vi "Automatic Teller Machine (ATM) SM based events.vi"() -> ()   [LabVIEW 2016]
doc: "This is the main VI of the ATM Machine simulation. This VI is developed using the design patterrn of Event based state machine."
uses:
  Controls/states.ctl
  Controls/Transaction Status.ctl
  Controls/UI Controls.ctl
  Controls/Module Data.ctl
  Controls/ATM Messages.ctl
  Controls/User Input Data.ctl
panel:
  in  "Module Data":T1={"UI Controls"={"ATM Messages"=refnum, "User Input"=refnum, "Right Buttons"=refnum, "Right Menu"=refnum, "Left Buttons"=refnum, "Left Menu"=refnum, "Card Simulator"=refnum, "Enter"=refnum}, "ATM Messages 2"={"Session terminate message"="Your session has been terminated\ndue to inactivity or menu selection.\nPlease take your card\n\nGoodbye!", "Welcome message"="Welcome to Acme bank.\nPlease insert your card\nand enter your account\nnumber in the User Input.\n\nPress Enter (E) when done.", "Deposit Message"="Please enter amount to deposit and press\nEnter (E) when done.", "Deposit Complete Message"="$ (Amount) Deposited", "Withdrawal Message"="Please enter amount to withdraw and press\nEnter (E) when done.", "Withdrawal Complete Message"="$ (Amount) Withdrawn", "Balance Inquiry Message"="Your Balance Is:\n$ (Balance amount from file)", "Account verification failed message"="Account information incorrect\nPlease Re-Enter Account Number.\nPress Enter (E) when done.", "Withdrawal failed message"="Insufficient funds in account\nplease check your balance\nand try again", "Card Inserted"="Card Inserted", "Main Menu message"="Welcome to Acme bank.\nFirst name, last Name (from file)\n\nplease select transaction\nby using the buttons."}, "User Input"="", "ATM Messages"="", "Acc. file path"=path "", "Accounts Data"=[], "User Input Data"={"Account No"="", "Amount"="", "Activity"=enum."Fast Cash $50"}, "Message"=""}
  in  "Enter":bool
  in  "User Input":string
  in  "Right Buttons":T6
  out "Right Menu":T7
  in  "Left Buttons":T6
  out "Left Menu":T7
  in  "Card Simulator":bool
  out "ATM Messages":string
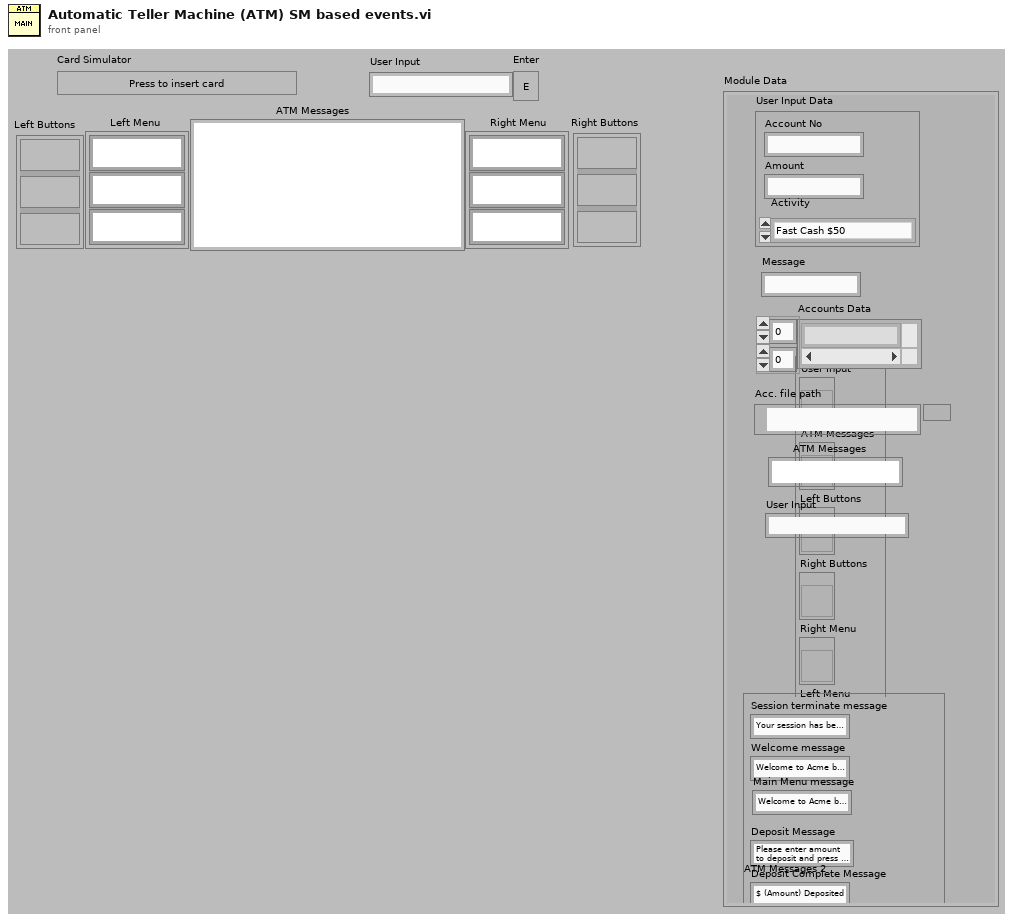
[diagram p1: front panel]
types:
  T1 = typedef "Module Data.ctl" = cluster{"UI Controls":T2, "ATM Messages 2":T3, "User Input":string, "ATM Messages":string, "Acc. file path":path, "Accounts Data":string[][], "User Input Data":T4, "Message":string}
  T2 = typedef "UI Controls.ctl" = cluster{"ATM Messages":refnum<vi>, "User Input":refnum<vi>, "Right Buttons":refnum<vi>, "Right Menu":refnum<vi>, "Left Buttons":refnum<vi>, "Left Menu":refnum<vi>, "Card Simulator":refnum<vi>, "Enter":refnum<vi>}
  T3 = typedef "ATM Messages.ctl" = cluster{"Session terminate message":string, "Welcome message":string, "Deposit Message":string, "Deposit Complete Message":string, "Withdrawal Message":string, "Withdrawal Complete Message":string, "Balance Inquiry Message":string, "Account verification failed message":string, "Withdrawal failed message":string, "Card Inserted":string, "Main Menu message":string}
  T4 = typedef "User Input Data.ctl" = cluster{"Account No":string, "Amount":string, "Activity":T5}
  T5 = typedef "Transaction Status.ctl" = enum16{"Fast Cash $50", "Withdrawal?", "Deposit?", "Account Number?"}
  T6 = cluster{"Func Button":bool, "Func Button 2":bool, "Func Button 3":bool}
  T7 = cluster{"RFS String":string, "RFS String 2":string, "RFS String 3":string}
  T8 = typedef "states.ctl" = enum16{"Deposit", "Enter Value", "Update Acc Number", "Make Correction in Acc No", "Wait for transaction", "Compare Account", "Read Accounts File", "Enter Account Number", "Wait for event", "Exit", "Initialize", "Insert ATM Card"}
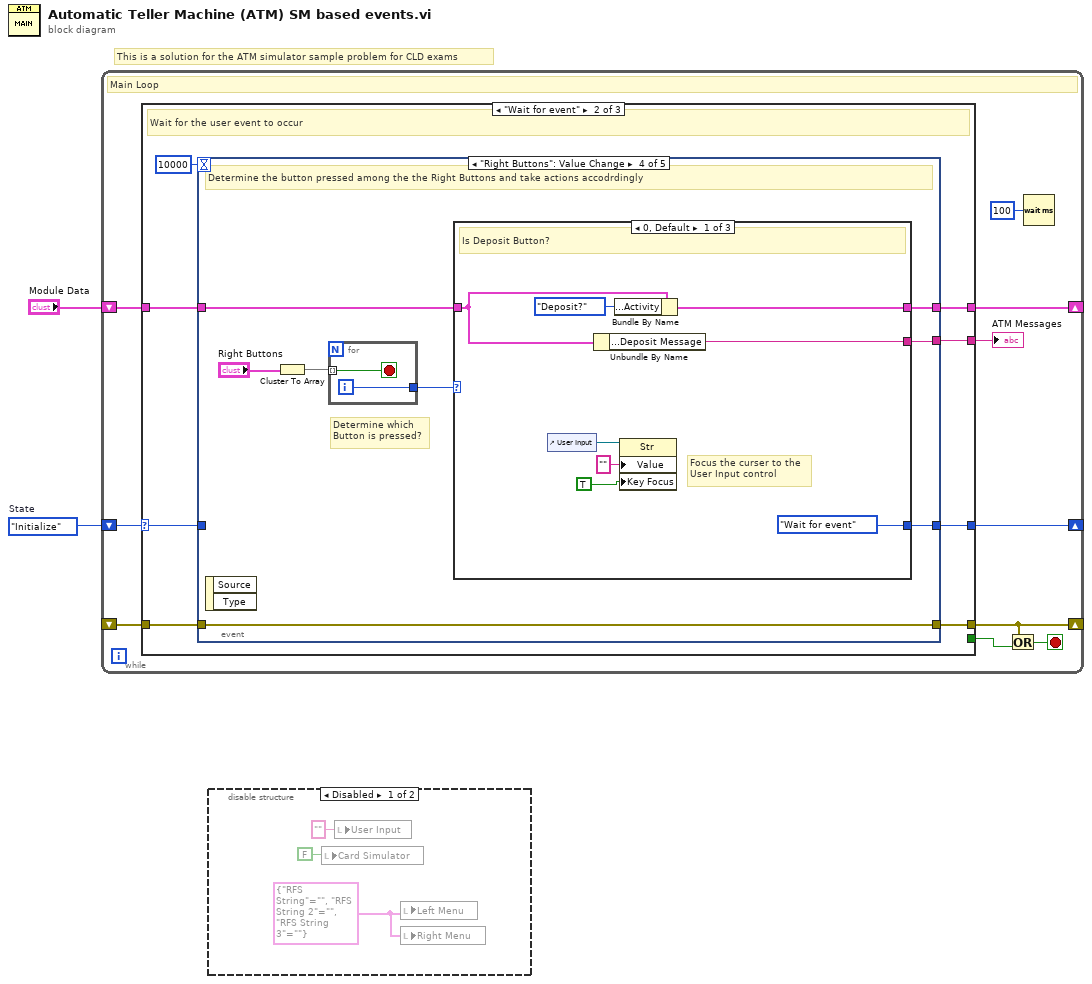
[diagram p0: block diagram]
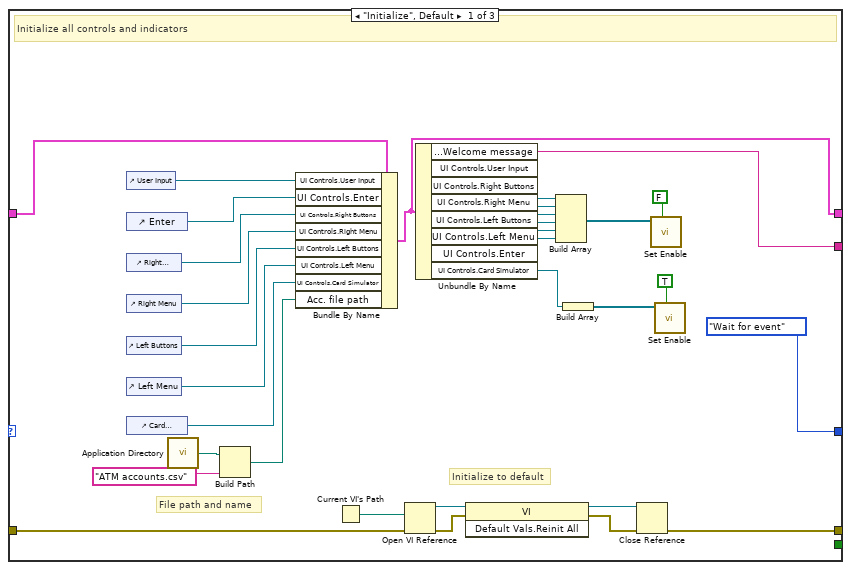
[diagram p3: hidden frame]
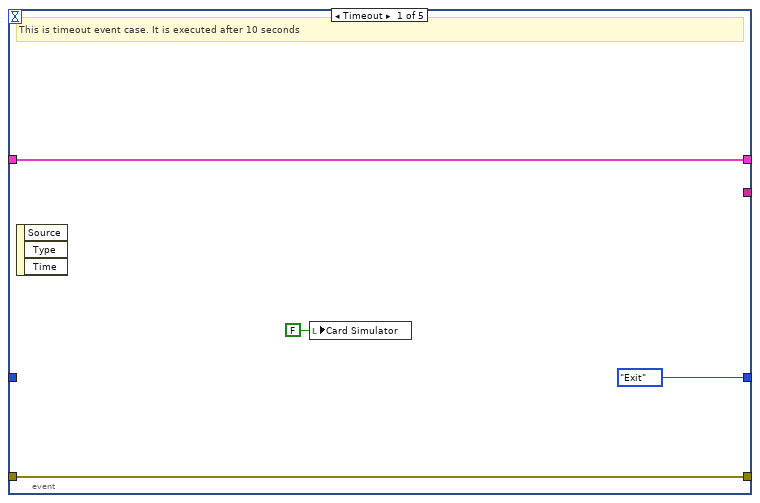
[diagram p4: hidden frame]
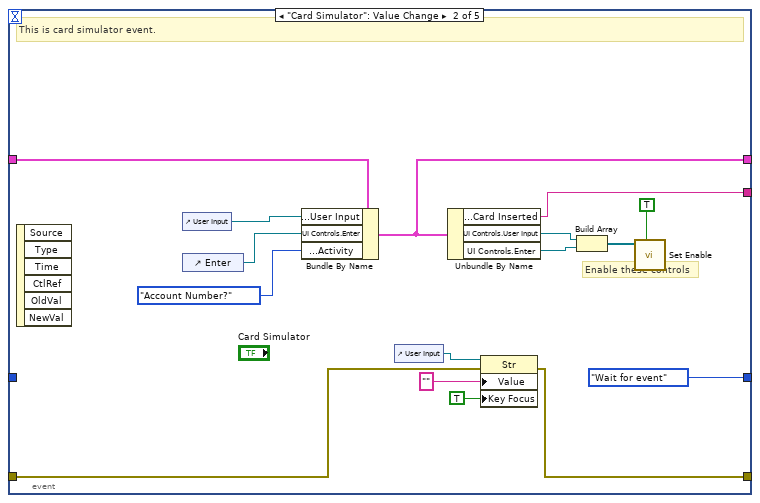
[diagram p5: hidden frame]
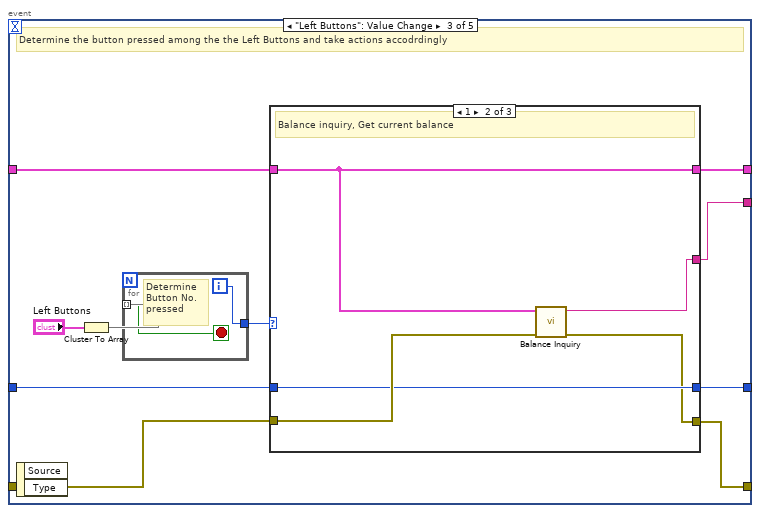
[diagram p6: hidden frame]
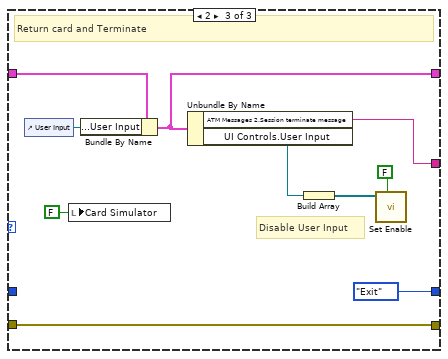
[diagram p8: hidden frame]
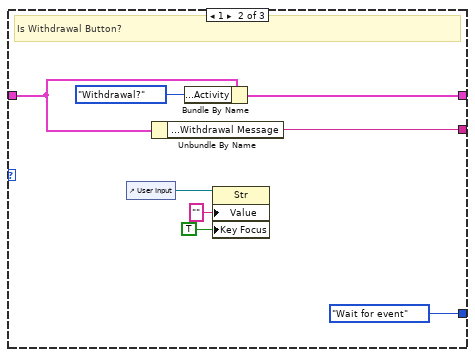
[diagram p9: hidden frame]
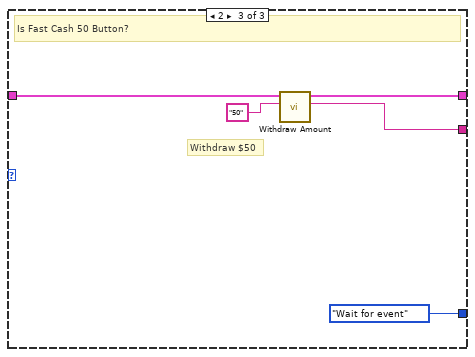
[diagram p10: hidden frame]
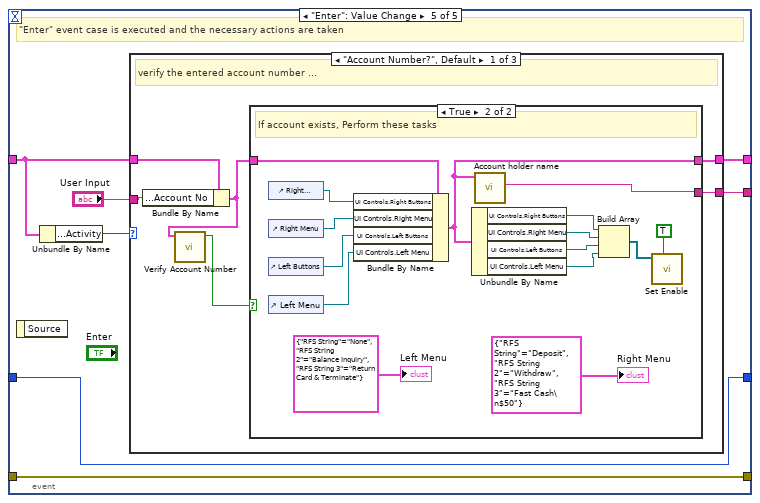
[diagram p11: hidden frame]
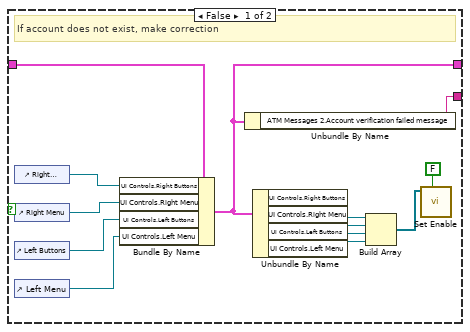
[diagram p12: hidden frame]
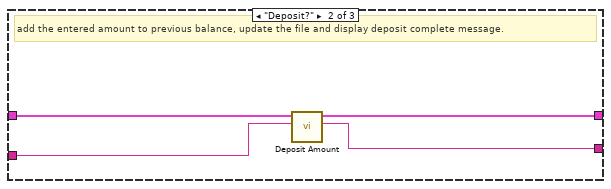
[diagram p13: hidden frame]
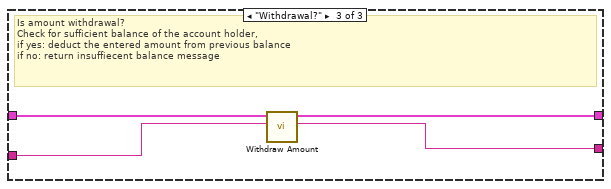
[diagram p14: hidden frame]
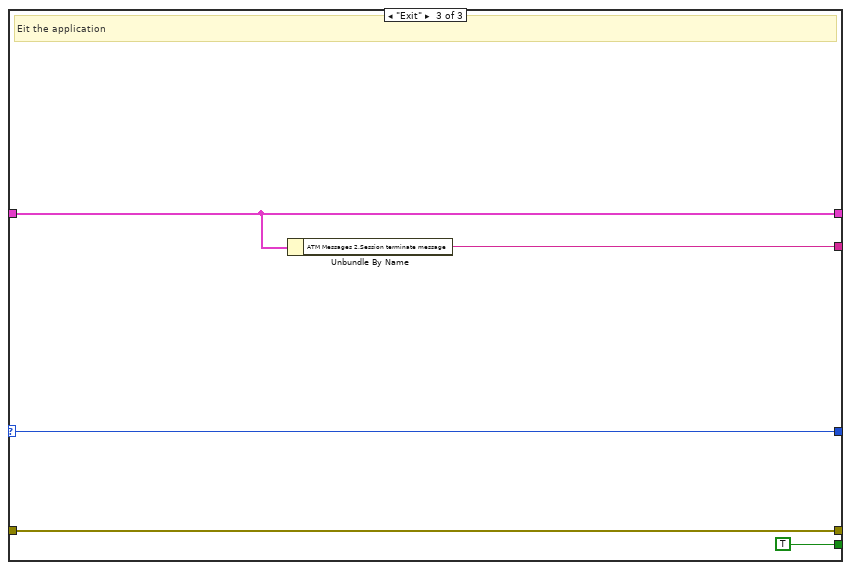
[diagram p15: hidden frame]
diagram:
  w1 = states."Initialize"  # State
  # "This is a solution for the ATM simulator sample problem for CLD exams"
  n1 = while {
    shift-right: [w12] -> _
    shift-left: "Module Data" -> [w11]
    shift-right: [w9] -> _
    shift-left: w1 -> [w10]
    shift-right: [w5] -> _
    shift-left: _ -> [w8]
    stop <- w3 stop-if-true
    # "Main Loop"
    n2 = case shown="\"Wait for event\"" w10 {
      selector: w10 -> [_ w49 w187]
      tunnel: [w28 w48 w183] -> w7
      tunnel: w11 -> [w33 w51 w184]
      tunnel: [w20 w45 w184] -> w12
      tunnel: [states."Wait for event" ("States") w50 w187] -> w9
      tunnel: [_ _ TRUE] -> w4
      tunnel: w8 -> [w17 w47 w185]
      tunnel: [w14 w46 w185] -> w5
      frame "Initialize", Default {
        # "Initialize to default"
        # "File path and name"
        # "Initialize all controls and indicators"
        n3 = control-ref of="User Input"() -> (w44:refnum<vi>)
        n4 = control-ref of="Enter"() -> (w43:refnum<vi>)
        n5 = control-ref of="Right Buttons"() -> (w42:refnum<vi>)
        n6 = control-ref of="Right Menu"() -> (w41:refnum<vi>)
        n7 = control-ref of="Left Buttons"() -> (w40:refnum<vi>)
        n8 = control-ref of="Left Menu"() -> (w39:refnum<vi>)
        n9 = control-ref of="Card Simulator"() -> (w25:refnum<vi>)
        n10 = call <vilib>:"Application Directory.vi"() -> ("Application Directory"=w23:path)
        n11 = Build Path(base path=w23, name or relative path="ATM accounts.csv") -> (appended path=w21:path)
        n12 = Bundle By Name(cluster=w33, "UI Controls.User Input"=w44, "UI Controls.Enter"=w43, "UI Controls.Right Buttons"=w42, "UI Controls.Right Menu"=w41, "UI Controls.Left Buttons"=w40, "UI Controls.Left Menu"=w39, "UI Controls.Card Simulator"=w25, "Acc. file path"=w21) -> (w20:T1)
        n13 = Current VI's Path() -> (path=w13:path)
        n14 = Open VI Reference(vi path=w13, error in (no error)=w17) -> (vi reference=w19:refnum<vi>, error out=w16:errorcluster)  [unwired: 4 in]
        n15 = Unbundle By Name(w20) -> ("ATM Messages 2.Welcome message"=w28:string, "UI Controls.User Input"=w38:refnum<vi>, "UI Controls.Right Buttons"=w37:refnum<vi>, "UI Controls.Right Menu"=w36:refnum<vi>, "UI Controls.Left Buttons"=w35:refnum<vi>, "UI Controls.Left Menu"=w34:refnum<vi>, "UI Controls.Enter"=w32:refnum<vi>, "UI Controls.Card Simulator"=w29:refnum<vi>)
        n16 = invoke class="VI" method="Default Vals.Reinit All"(reference=w19, error in=w16) -> (reference out=w18:refnum<vi>, error out=w15:errorcluster)  [unwired: 1 in, 1 out]
        n17 = Build Array(w38, w37, w36, w35, w34, w32) -> (w31:refnum<vi>[])
        n18 = Build Array(w29) -> (w30:refnum<vi>[])
        n19 = Close Reference(reference=w18, error in (no error)=w15) -> (error out=w14:errorcluster)
        n20 = call "Set Enable.vi"("Enable?"=FALSE, "UI Controls"=w31) -> ()  [unwired: 10 in]
        n21 = call "Set Enable.vi"("Enable?"=TRUE, "UI Controls"=w30) -> ()  [unwired: 10 in]
      }
      frame "Wait for event" {
        # "Wait for the user event to occur"
        n22 = event shown="[3] \"Right Buttons\": Value Change" {
          selector: _ -> [_ _ _ _ _]
          dyn-events: _ -> [_ _ _ _ _]
          timeout: 10000 -> [_ _ _ _ _]
          tunnel: w51 -> [w55 w69 w79 w106 w136]
          tunnel: [states."Exit" ("States") states."Wait for event" ("States") w75 w103 w135] -> w50
          tunnel: w49 -> [_ _ w74 _ w135]
          tunnel: [_ w64 w77 w105 w134] -> w48
          tunnel: w47 -> [w54 w57 w78 w110 w137]
          tunnel: [w54 w58 w73 w110 w137] -> w46
          tunnel: [w55 w62 w76 w104 w139] -> w45
          event Timeout {
            # "This is timeout event case. It is executed after 10 seconds"
            n23 = event-data() -> ()  [unwired: 1 in, 3 out]
            n24 = local write "Card Simulator"(FALSE ("Card Simulator")) -> ()
          }
          event "Card Simulator": Value Change {
            # "Enable these controls"
            # "This is card simulator event."
            n25 = event-data() -> ()  [unwired: 1 in, 6 out]
            n26 = control-ref of="User Input"() -> (w72:refnum<vi>)
            n27 = control-ref of="Enter"() -> (w71:refnum<vi>)
            n28 = Bundle By Name(cluster=w69, "UI Controls.User Input"=w72, "UI Controls.Enter"=w71, "User Input Data.Activity"=Transaction_Status."Account Number?" ("User Input Data.Transactions")) -> (w62:T1)
            n29 = control-ref of="User Input"() -> (w61:refnum<vi>)
            n30 = Unbundle By Name(w62) -> ("ATM Messages 2.Card Inserted"=w64:string, "UI Controls.User Input"=w68:refnum<vi>, "UI Controls.Enter"=w67:refnum<vi>)
            n31 = property class="Str"(reference=w61, error in=w57, "Value"="", "Key Focus"=TRUE) -> (error out=w58:errorcluster)  [unwired: 1 out]
            n32 = Build Array(w68, w67) -> (w66:refnum<vi>[])
            n33 = call "Set Enable.vi"("Enable?"=TRUE, "UI Controls"=w66) -> ()  [unwired: 10 in]
          }
          event "Left Buttons": Value Change {
            # "Determine the button pressed among the the Left Buttons and take actions accodrdingly"
            n34 = event-data() -> ()  [unwired: 1 in, 2 out]
            n35 = Cluster To Array(cluster="Left Buttons") -> (array=w81:bool[])
            n36 = for {
              tunnel: w81 -> [w84] mode=indexing
              tunnel: [w83] -> w80
              i -> [w83]
              stop <- w84 stop-if-true
              # "Determine\nButton No. \npressed"
            }
            n37 = case shown="1" w80 {
              tunnel: w79 -> [w87 w90 w101]
              tunnel: w78 -> [w85 w92 w98]
              tunnel: [_ w91 w93] -> w77
              tunnel: [w87 w90 w97] -> w76
              tunnel: [w86 w89 states."Exit" ("States")] -> w75
              tunnel: w74 -> [w86 w89 _]
              tunnel: [w85 w88 w98] -> w73
              frame 0, Default {
                # "Do nothing, this button is for\nfuture use."
              }
              frame 1 {
                # "Balance inquiry, Get current balance"
                n38 = call "Balance Inquiry.vi"("error in (no error)"=w92, "Module Data"=w90) -> ("error out"=w88:errorcluster, "Balance"=w91:string)  [unwired: 8 in]
              }
              frame 2 {
                # "Disable User Input"
                # "Return card and Terminate"
                n39 = control-ref of="User Input"() -> (w100:refnum<vi>)
                n40 = local write "Card Simulator"(FALSE ("Card Simulator")) -> ()
                n41 = Bundle By Name(cluster=w101, "UI Controls.User Input"=w100) -> (w97:T1)
                n42 = Unbundle By Name(w97) -> ("ATM Messages 2.Session terminate message"=w93:string, "UI Controls.User Input"=w96:refnum<vi>)
                n43 = Build Array(w96) -> (w95:refnum<vi>[])
                n44 = call "Set Enable.vi"("Enable?"=FALSE, "UI Controls"=w95) -> ()  [unwired: 10 in]
              }
            }
          }
          event "Right Buttons": Value Change {
            # "Determine which\nButton is pressed?"
            # "Determine the button pressed among the the Right Buttons and take actions accodrdingly"
            n45 = event-data() -> ()  [unwired: 1 in, 2 out]
            n46 = Cluster To Array(cluster="Right Buttons") -> (array=w108:bool[])
            n47 = for {
              tunnel: w108 -> [w132] mode=indexing
              tunnel: [w133] -> w107
              i -> [w133]
              stop <- w132 stop-if-true
            }
            n48 = case shown="0, Default" w107 {
              tunnel: w106 -> [w116 w124 w130]
              tunnel: [w117 w125 w127] -> w105
              tunnel: [w115 w123 w128] -> w104
              tunnel: [states."Wait for event" ("States") states."Wait for event" ("States") states."Wait for event" ("States")] -> w103
              frame 0, Default {
                # "Focus the curser to the\nUser Input control"
                # "Is Deposit Button?"
                n49 = control-ref of="User Input"() -> (w114:refnum<vi>)
                n50 = Unbundle By Name(w116) -> ("ATM Messages 2.Deposit Message"=w117:string)
                n51 = Bundle By Name(cluster=w116, "User Input Data.Activity"=Transaction_Status."Deposit?") -> (w115:T1)
                n52 = property class="Str"(reference=w114, "Value"="", "Key Focus"=TRUE) -> ()  [unwired: 1 in, 2 out]
              }
              frame 1 {
                # "Is Withdrawal Button?"
                n53 = control-ref of="User Input"() -> (w121:refnum<vi>)
                n54 = Unbundle By Name(w124) -> ("ATM Messages 2.Withdrawal Message"=w125:string)
                n55 = Bundle By Name(cluster=w124, "User Input Data.Activity"=Transaction_Status."Withdrawal?" ("Transactions")) -> (w123:T1)
                n56 = property class="Str"(reference=w121, "Value"="", "Key Focus"=TRUE) -> ()  [unwired: 1 in, 2 out]
              }
              frame 2 {
                # "Withdraw $50"
                # "Is Fast Cash 50 Button?"
                n57 = call "Withdraw Amount.vi"("User Input"="50", "Module Data in"=w130) -> ("Withdrawal Complete Message"=w127:string, "Module Data out"=w128:T1)  [unwired: 8 in]
              }
            }
          }
          event "Enter": Value Change {
            # "\"Enter\" event case is executed and the necessary actions are taken"
            n58 = event-data() -> ()  [unwired: 1 in, 1 out]
            n59 = Unbundle By Name(w136) -> ("User Input Data.Activity"=w140:T5)
            n60 = case shown="\"Account Number?\", Default" w140 {
              tunnel: w136 -> [w144 w176 w180]
              tunnel: [w143 w175 w182] -> w139
              tunnel: "User Input" -> [w146 w177 w179]
              tunnel: [w142 w178 w181] -> w134
              frame "Account Number?", Default {
                # "verify the entered account number ..."
                n61 = Bundle By Name(cluster=w144, "User Input Data.Account No"=w146) -> (w141:T1)
                n62 = call "Verify Account Number.vi"("Module Data"=w141) -> ("Is account?"=w145:bool)  [unwired: 6 in, 4 out]
                n63 = case shown="True" w145 {
                  tunnel: [w148 w161] -> w143
                  tunnel: w141 -> [w149 w174]
                  tunnel: [w159 w160] -> w142
                  frame False {
                    # "If account does not exist, make correction"
                    n64 = control-ref of="Right Buttons"() -> (w152:refnum<vi>)
                    n65 = control-ref of="Right Menu"() -> (w151:refnum<vi>)
                    n66 = control-ref of="Left Buttons"() -> (w150:refnum<vi>)
                    n67 = control-ref of="Left Menu"() -> (w147:refnum<vi>)
                    n68 = Bundle By Name(cluster=w149, "UI Controls.Right Buttons"=w152, "UI Controls.Right Menu"=w151, "UI Controls.Left Buttons"=w150, "UI Controls.Left Menu"=w147) -> (w148:T1)
                    n69 = Unbundle By Name(w148) -> ("ATM Messages 2.Account verification failed message"=w159:string)
                    n70 = Unbundle By Name(w148) -> ("UI Controls.Right Buttons"=w158:refnum<vi>, "UI Controls.Right Menu"=w157:refnum<vi>, "UI Controls.Left Buttons"=w156:refnum<vi>, "UI Controls.Left Menu"=w155:refnum<vi>)
                    n71 = Build Array(w158, w157, w156, w155) -> (w154:refnum<vi>[])
                    n72 = call "Set Enable.vi"("Enable?"=FALSE, "UI Controls"=w154) -> ()  [unwired: 10 in]
                  }
                  frame True {
                    # "If account exists, Perform these tasks"
                    n73 = control-ref of="Right Buttons"() -> (w173:refnum<vi>)
                    n74 = control-ref of="Right Menu"() -> (w172:refnum<vi>)
                    n75 = control-ref of="Left Buttons"() -> (w171:refnum<vi>)
                    n76 = control-ref of="Left Menu"() -> (w170:refnum<vi>)
                    n77 = Bundle By Name(cluster=w174, "UI Controls.Right Buttons"=w173, "UI Controls.Right Menu"=w172, "UI Controls.Left Buttons"=w171, "UI Controls.Left Menu"=w170) -> (w161:T1)
                    n78 = Unbundle By Name(w161) -> ("UI Controls.Right Buttons"=w167:refnum<vi>, "UI Controls.Right Menu"=w166:refnum<vi>, "UI Controls.Left Buttons"=w165:refnum<vi>, "UI Controls.Left Menu"=w164:refnum<vi>)
                    n79 = call "Account holder name.vi"("Module Data in"=w161) -> ("Withdrawal Complete Message"=w160:string)  [unwired: 10 in]
                    n80 = Build Array(w167, w166, w165, w164) -> (w163:refnum<vi>[])
                    n81 = call "Set Enable.vi"("Enable?"=TRUE, "UI Controls"=w163) -> ()  [unwired: 10 in]
                    "Left Menu" <- T7 {"RFS String"="None", "RFS String 2"="Balance Inquiry", "RFS String 3"="Return Card & Terminate"} ("Left Menu")
                    "Right Menu" <- T7 {"RFS String"="Deposit", "RFS String 2"="Withdraw", "RFS String 3"="Fast Cash\n$50"} ("Right Menu")
                  }
                }
              }
              frame "Deposit?" {
                # "add the entered amount to previous balance, update the file and display deposit complete message."
                n82 = call "Deposit Amount.vi"("User Input"=w177, "Module Data in"=w176) -> ("Deposit Complete Message"=w178:string, "Module Data out"=w175:T1)  [unwired: 8 in]
              }
              frame "Withdrawal?" {
                # "Is amount withdrawal?\nCheck for sufficient balance of the account holder, \nif yes: deduct the entered amount from previous balance\nif no: return insuffiecent balance message"
                n83 = call "Withdraw Amount.vi"("User Input"=w179, "Module Data in"=w180) -> ("Withdrawal Complete Message"=w181:string, "Module Data out"=w182:T1)  [unwired: 8 in]
              }
            }
          }
        }
      }
      frame "Exit" {
        # "Eit the application"
        n84 = Unbundle By Name(w184) -> ("ATM Messages 2.Session terminate message"=w183:string)
      }
    }
    "ATM Messages" <- w7
    n85 = Or(x=w5, y=w4) -> (x .or. y?=w3:bool)
    n86 = Wait (ms)(milliseconds to wait=u32 100) -> ()  [unwired: 1 out]
  }
  n87 = disable-structure shown="Disabled" {
    frame Disabled {
      w189 = T7 {"RFS String"="", "RFS String 2"="", "RFS String 3"=""} ("Left Menu")
      n88 = local write "Card Simulator"(FALSE ("Card Simulator")) -> ()
      n89 = local write "User Input"("" ("User Input")) -> ()
      n90 = local write "Left Menu"(w189) -> ()
      n91 = local write "Right Menu"(w189) -> ()
    }
    frame Enabled {
    }
  }
